vi "SaveCalibrationResults.vi"(8 "error in":errorcluster, 10 "correctedFreqList":T1(array[cluster]), 11 "file path calibration results":path=path "C:/PRUEF/MIC_EOL_TS2016/Sourcecode/ProjectSourcecode/Config Files/calibrationResults.txt") -> (0 "error out":errorcluster)   [LabVIEW 2018]
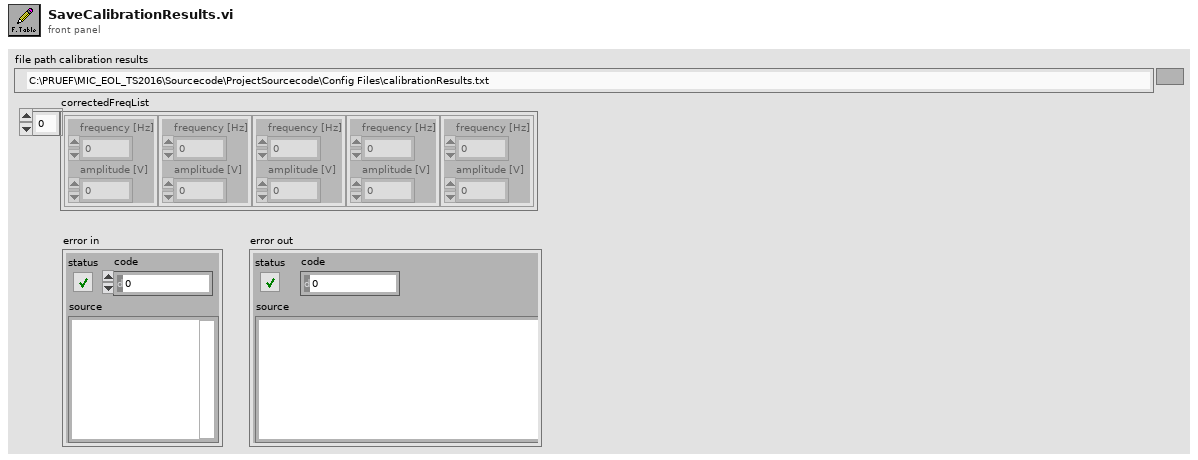
[diagram p1: front panel]
types:
  T1 = cluster{"frequency [Hz]":dbl, "amplitude [V]":dbl}[]
  T2 = enum16{"open", "replace", "create", "open or create", "replace or create", "replace or create with confirmation"}
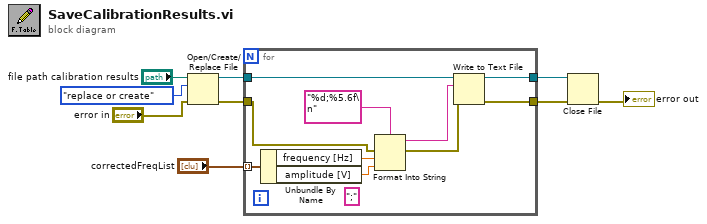
[diagram p0: block diagram]
diagram:
  n1 = Open/Create/Replace File(file path (use dialog)="file path calibration results", error in="error in", operation (0:open)=T2."replace or create") -> (refnum out=w8:refnum<file>, error out=w7:errorcluster)  [unwired: 3 in, 1 out]
  n2 = for {
    tunnel: "correctedFreqList" -> [w19] mode=indexing
    tunnel: w8 -> [w16]
    tunnel: w7 -> [w13]
    tunnel: [w12] -> w6
    tunnel: [w11] -> w5
    (unwired) ";" ("string")
    n3 = Unbundle By Name(w19) -> ("frequency [Hz]"=w17:dbl, "amplitude [V]"=w10:dbl)
    n4 = Format Into String(format string="%d;%5.6f\n", error in=w13, w17, w10) -> (resulting string=w15:string, error out=w14:errorcluster)  [unwired: 1 in]
    n5 = Write to Text File(file (use dialog)=w16, text=w15, error in=w14) -> (refnum out=w12:refnum<file>, error out=w11:errorcluster)  [unwired: 1 in, 1 out]
  }
  n6 = Close File(refnum=w6, error in=w5) -> (error out=→"error out":errorcluster)  [unwired: 1 out]
